vi "OffsetData.vi"() -> ()   [LabVIEW 2018]
panel:
  out "New Dynamic Load Force":dbl
  out "New Static Load Force":dbl
  out "New Grip Force":dbl
  out "New Elbow Angle":dbl
  in  "Elbow Angle":dbl
  in  "Grip Force":dbl
  in  "Dynamic Load Force":dbl
  in  "Static Load Force":dbl
  # "Futek Sensor"
  # "HX711 Sensor"
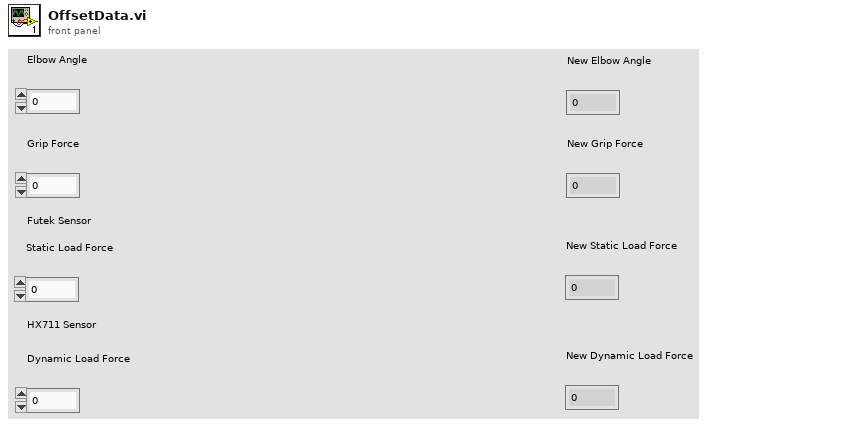
[diagram p1: front panel]
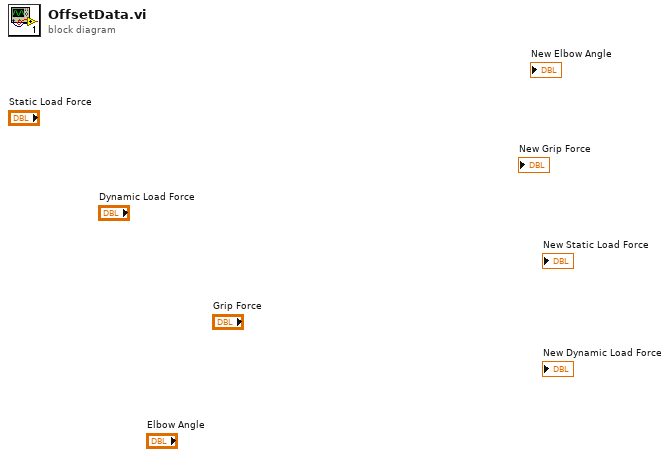
[diagram p0: block diagram]
diagram:
